vi "BC-Clip-Ball_Api.vi"(8 "Error In":errorcluster, 11 "校正微動位置":enum16{"雙邊", "オ", "右"}(ring)) -> (0 "Error Out":errorcluster)   [LabVIEW 2019]
uses:
  <vilib>/Platform/TimedLoop/XDataNode/timing_clust.ctl
  <vilib>/Platform/TimedLoop/XDataNode/nitl_modes.ctl
  <vilib>/Platform/TimedLoop/XDataNode/wakeup.ctl
  <vilib>/platform/TimedLoop/XDataNode/XDataNode.xnode
  <vilib>/Platform/TimedLoop/XDataNode/XDNodeRunTimeDep.lvlib
panel:
  in  "Stop":bool
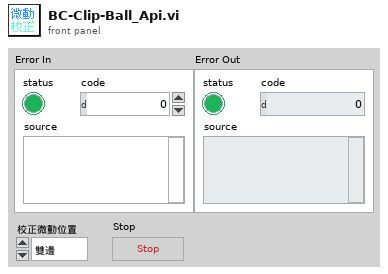
[diagram p1: front panel]
types:
  T1 = typedef "XDNodeRunTimeDep.lvlib/timing_clust.ctl" = cluster{"Expected End [f-1]":u64, "Actual End [f-1]":u64, "Finished Late? [f-1]":bool, "Expected End [i-1]":u64, "Actual End [i-1]":u64, "Finished Late? [i-1]":bool, "Expected Start [i]":u64, "Actual Start [i]":u64, "Expected Start [f]":u64, "Actual Start [f]":u64, "Source Name":string, "Structure Name":string, "Period":i64, "Deadline":i64, "Offset":i64, "Start":i64, "Priority":i32, "Timeout":i32, "Mode":T2, "Wakeup Reason":T3, "Error":errorcluster, "Source Type":string, "Secondary Source Type":string, "Global End Time":u64, "Global Start Time":u64, "Frame Duration":u64, "Iteration Duration":u64, "Assigned CPU":i32, "I/O Scan Engine Mode":u32}
  T2 = typedef "XDNodeRunTimeDep.lvlib/nitl_modes.ctl" = enum32{"No Change", "Process missed periods, maintain original phase", "Discard missed periods, maintain original phase", "Process missed periods, ignore original phase", "Discard missed periods, ignore original phase"}
  T3 = typedef "XDNodeRunTimeDep.lvlib/wakeup.ctl" = enum32{"Normal", "Aborted", "Asynchronous wakeup", "Timing source error", "Timed loop error", "Timeout"}
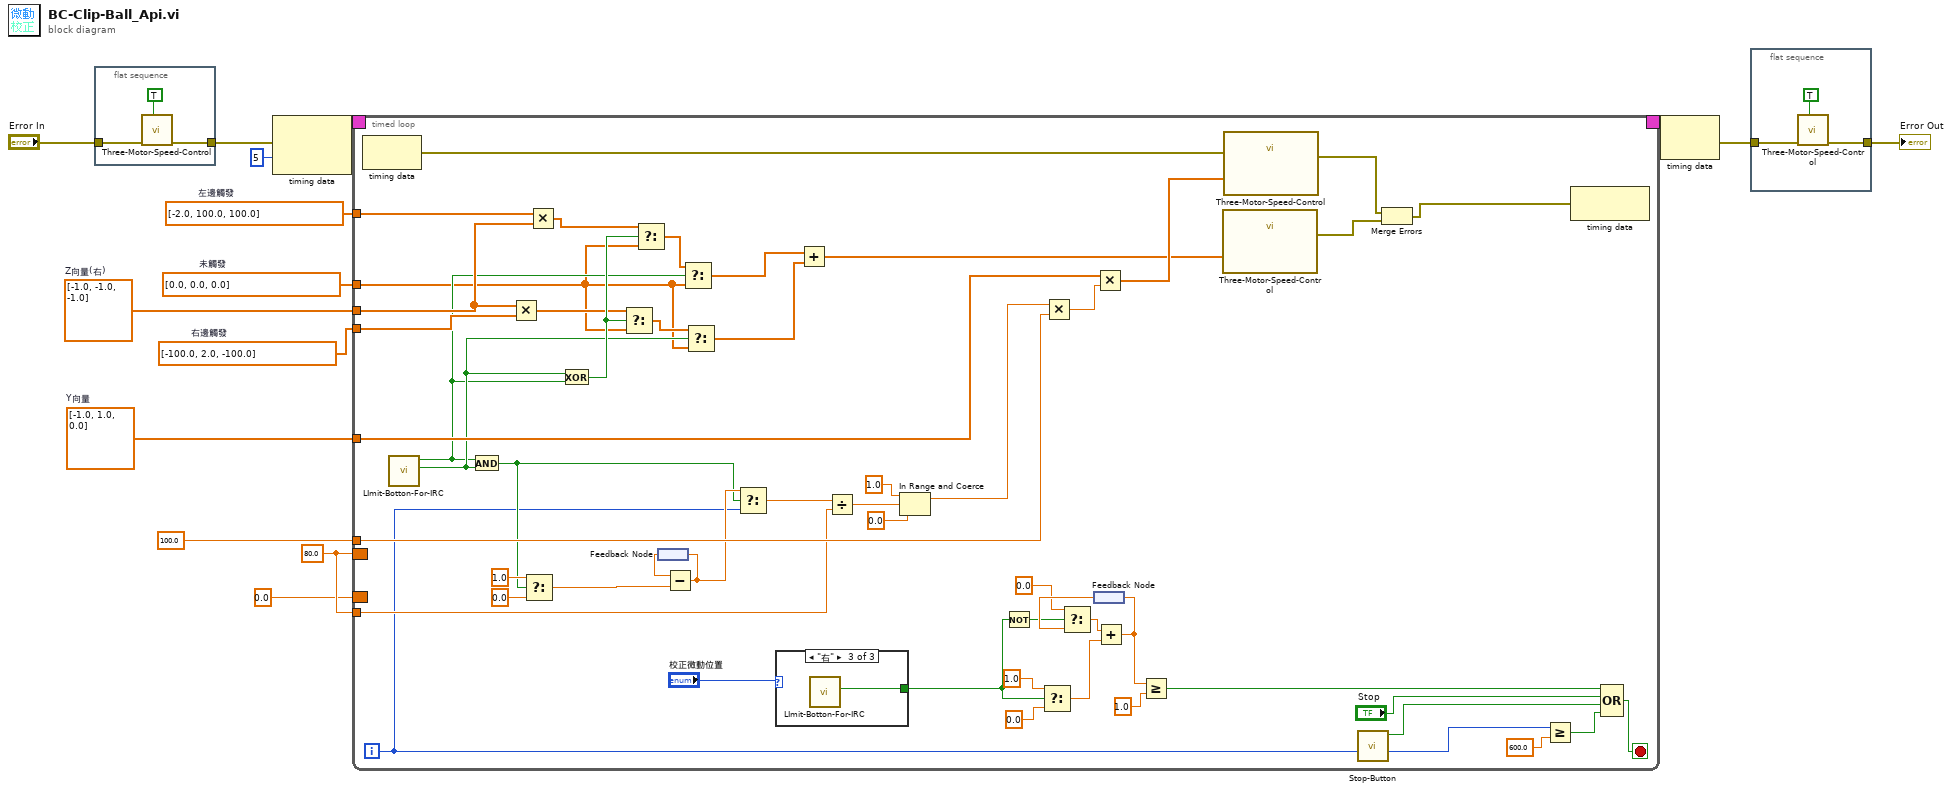
[diagram p0: block diagram]
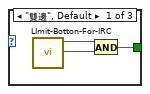
[diagram p2: hidden frame]
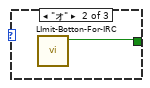
[diagram p3: hidden frame]
diagram:
  w4 = dbl[] [0.0, 0.0, 0.0]  # 未觸發
  w6 = dbl[] [-100.0, 2.0, -100.0]  # 右邊觸發
  w5 = dbl[] [-2.0, 100.0, 100.0]  # 左邊觸發
  w7 = dbl[] [-1.0, -1.0, -1.0]  # Z向量(右)
  w11 = 80.0
  w10 = dbl[] [-1.0, 1.0, 0.0]  # Y向量
  n1 = flat-sequence {
    tunnel: "Error In" -> [w17]
    tunnel: [w16] -> w9
    frame #0 {
      n2 = call "Three-Motor-Speed-Control.vi"("Reset"=TRUE, "Error In"=w17) -> ("Error Out"=w16:errorcluster)  [unwired: 9 in]
    }
  }
  n3 = node-c288(w9, i64 5 ("Period")) -> (w15:T1)
  n4 = timed-loop {
    timing: w15 -> [_]
    timing-out: [_] -> w14
    tunnel: 100.0 -> [w66]
    border: w11 -> [_]
    tunnel: w11 -> [w59]
    tunnel: w10 -> [w54]
    tunnel: w7 -> [w50]
    tunnel: w6 -> [w52]
    tunnel: w5 -> [w51]
    tunnel: w4 -> [w34]
    border: 0.0 -> [_]
    i -> [w19]
    stop <- w69 stop-if-true
    n5 = node-c288() -> (w70:errorcluster)  [unwired: 1 in]
    n6 = call "LImit-Botton-For-IRC.vi"() -> ("微動觸發(右)?"=w36:bool, "微動觸發(左)?"=w35:bool)  [unwired: 9 in, 1 out]
    n7 = And(x=w35, y=w36) -> (x .and. y?=w41:bool)
    n8 = Multiply(x=w50, y=w52) -> (x*y=w37:dbl[])
    n9 = Select(t=1.0, s=w41, f=0.0) -> (s? t:f=w64:dbl)
    n10 = Multiply(x=w51, y=w50) -> (x*y=w38:dbl[])
    n11 = Exclusive Or(1:w35, 2:w36) -> (0:w39:bool)
    n12 = Select(t=w37, s=w39, f=w34) -> (s? t:f=w40:dbl[])
    n13 = Select(t=w38, s=w39, f=w34) -> (s? t:f=w42:dbl[])
    n14 = feedback #1() -> (w63:dbl)
    n15 = Subtract(x=w63, y=w64) -> (x-y=w62:dbl)
    n16 = feedback-in #1(w62) -> ()
    n17 = Select(t=w42, s=w35, f=w34) -> (s? t:f=w45:dbl[])
    n18 = Select(t=w40, s=w36, f=w34) -> (s? t:f=w44:dbl[])
    n19 = Select(t=w62, s=w41, f=w19) -> (s? t:f=w61:dbl)
    n20 = case shown="\"右\"" "校正微動位置" {
      tunnel: [w71 w74 w75] -> w23
      frame "雙邊", Default {
        n21 = call "LImit-Botton-For-IRC.vi"() -> ("微動觸發(右)?"=w72:bool, "微動觸發(左)?"=w73:bool)  [unwired: 9 in, 1 out]
        n22 = And(x=w73, y=w72) -> (x .and. y?=w71:bool)
      }
      frame "オ" {
        n23 = call "LImit-Botton-For-IRC.vi"() -> ("微動觸發(左)?"=w74:bool)  [unwired: 9 in, 2 out]
      }
      frame "右" {
        n24 = call "LImit-Botton-For-IRC.vi"() -> ("微動觸發(右)?"=w75:bool)  [unwired: 9 in, 2 out]
      }
    }
    n25 = Add(x=w45, y=w44) -> (x+y=w43:dbl[])
    n26 = Divide(x=w61, y=w59) -> (x/y=w58:dbl)
    n27 = In Range and Coerce(upper limit=1.0, x=w58, lower limit=0.0) -> (coerced(x)=w55:dbl)  [unwired: 1 out]
    n28 = Not(x=w23) -> (.not. x?=w28:bool)
    n29 = Select(t=1.0, s=w23, f=0.0) -> (s? t:f=w30:dbl)
    n30 = Multiply(x=w55, y=w66) -> (x*y=w53:dbl)
    n31 = feedback #2() -> (w29:dbl)
    n32 = Select(t=0.0, s=w28, f=w29) -> (s? t:f=w26:dbl)
    n33 = Multiply(x=w54, y=w53) -> (x*y=w49:dbl[])
    n34 = Add(x=w26, y=w30) -> (x+y=w25:dbl)
    n35 = feedback-in #2(w25) -> ()
    n36 = Greater Or Equal?(x=w25, y=1.0) -> (x >= y?=w22:bool)
    n37 = call "Three-Motor-Speed-Control.vi"("速度(秒/度)"=w43) -> ("Error Out"=w46:errorcluster)  [unwired: 10 in]
    n38 = call "Three-Motor-Speed-Control.vi"("Error In"=w70, "速度(秒/度)"=w49) -> ("Error Out"=w47:errorcluster)  [unwired: 9 in]
    n39 = call "Stop-Button.vi"() -> ("顯示按下?"=w67:bool)  [unwired: 10 in, 1 out]
    n40 = Merge Errors(w47, w46) -> (w48:errorcluster)
    n41 = Greater Or Equal?(x=w19, y=600.0) -> (x >= y?=w21:bool)
    n42 = node-c288(w48) -> ()  [unwired: 1 out]
    n43 = Compound Arithmetic op=OR(w22, "Stop", w67, w21) -> (w69:bool)
  }
  n44 = node-c288(w14) -> (w8:errorcluster)
  n45 = flat-sequence {
    tunnel: w8 -> [w82]
    tunnel: [w81] -> w1
    frame #0 {
      n46 = call "Three-Motor-Speed-Control.vi"("Reset"=TRUE, "Error In"=w82) -> ("Error Out"=w81:errorcluster)  [unwired: 9 in]
    }
  }
  "Error Out" <- w1
